vi "Next Bind (name).vi"(8 "error in (no error)":errorcluster, 10 "parameter name":string, 11 "SQL Statement in":refnum<class "SQL Statement.lvclass">) -> (0 "error out":errorcluster, 3 "SQL Statement out":refnum<class "SQL Statement.lvclass">)   [LabVIEW 2013, in "SQLiteSupport.lvlib" / "SQL Statement.lvclass"]
doc: "Sets the next parameter to be bound to, by its name. Name formats are ?NNN, :VVV, @VVV or $VVV where NNN are numeric digits and VVV are alphanumeric characters. Names are specified in the SQL statement."
uses:
  SQL Statement.lvclass
  SQL Statement.lvclass/SQL Statement.ctl
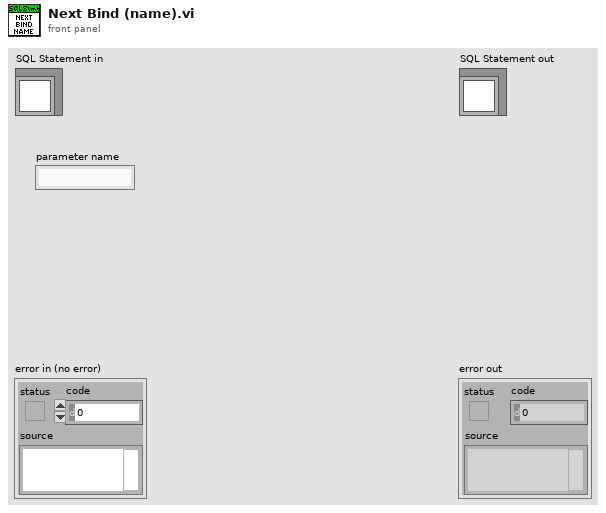
[diagram p1: front panel]
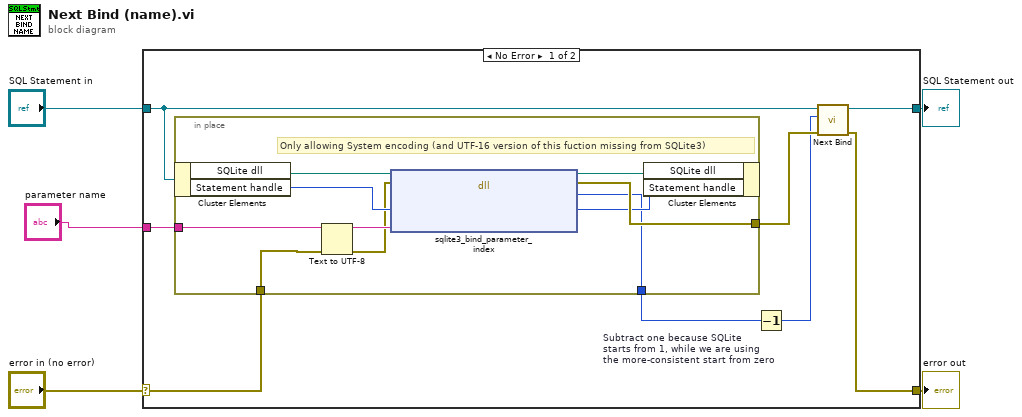
[diagram p0: block diagram]
diagram:
  n1 = case shown="No Error" "error in (no error)" {
    selector: "error in (no error)" -> [w13 w25]
    tunnel: [w9 w25] -> w4
    tunnel: [w11 w24] -> w2
    tunnel: "SQL Statement in" -> [w7 w24]
    tunnel: "parameter name" -> [w12 _]
    frame No Error {
      n2 = in-place {
        in-place-border: w13 -> [w23]
        in-place-border: w12 -> [w22]
        in-place-border: [w21] -> w10
        in-place-border: [w16] -> w6
        # "Only allowing System encoding (and UTF-16 version of this fuction missing from SQLite3)"
        n3 = in-place-cluster #1(w7) -> ("SQLite dll"=w20:path, "Statement handle"=w18:u64)
        n4 = Text to UTF-8(8:w23, 11:w22) -> (0:w14:errorcluster, 3:w15:string)
        n5 = dll-call lib="C:/LabVIEW_JDP/Support/SQLite/sqlite3.dll" fn="sqlite3_bind_parameter_index"(path in=w20, error in=w14, "Statement"=w18, "name"=w15) -> (path out=w19:path, error out=w21:errorcluster, "Paramter index"=w16:i32, "Statement"=w17:u64)  [unwired: 2 in]
        n6 = in-place-cluster #1("SQLite dll"=w19, "Statement handle"=w17) -> ()  [unwired: 1 out]
      }
      n7 = Decrement "Subtract one because SQLite\nstarts from 1, while we are using\nthe more-consistent start from zero"(x=w6) -> (x-1=w8:i32)
      n8 = call "Next Bind.vi"("error in (no error)"=w10, "Next Bind"=w8, "SQL Statement in"=w7) -> ("error out"=w9:errorcluster, "SQL Statement out"=w11:refnum<class "SQL Statement.lvclass">)  [unwired: 7 in]
    }
    frame Error {
    }
  }
  "error out" <- w4
  "SQL Statement out" <- w2
